vi "Exercice4Operations.vi"() -> ()   [LabVIEW 2018]
panel:
  in  "b":dbl(slide) scale=0.0..9.0
  in  "a":dbl
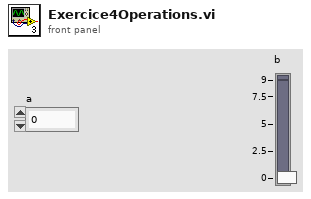
[diagram p1: front panel]
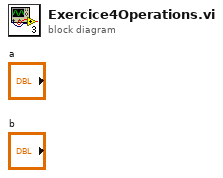
[diagram p0: block diagram]
diagram:
